vi "solar_visa VISA Query (Error).vi"(6 "ms Read Wait (0)":u32, 8 "error in (no error)":errorcluster, 9 "Bytes Expected (0 = 1024)":u32, 10 "Error Query (\"\" = No Query)":string, 11 "VISA Resource in":refnum<visa-resource-name>) -> (0 "error out":errorcluster, 3 "VISA Resource out":refnum<visa-resource-name>)   [LabVIEW 2018]
doc: "This queries instrument errors from the VISA session. By default, the error code integer is expected at the begining of the <b>Error Query</b> response (i.e \"+7: Invalid parameter...\"). To avoid an error lockout, the error query is limited to 100 errors. \nIf <b>Error in</b> contains a timeout error this clears the VISA buffer."
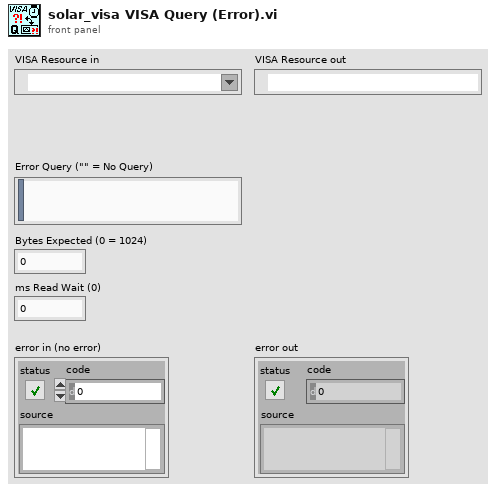
[diagram p1: front panel]
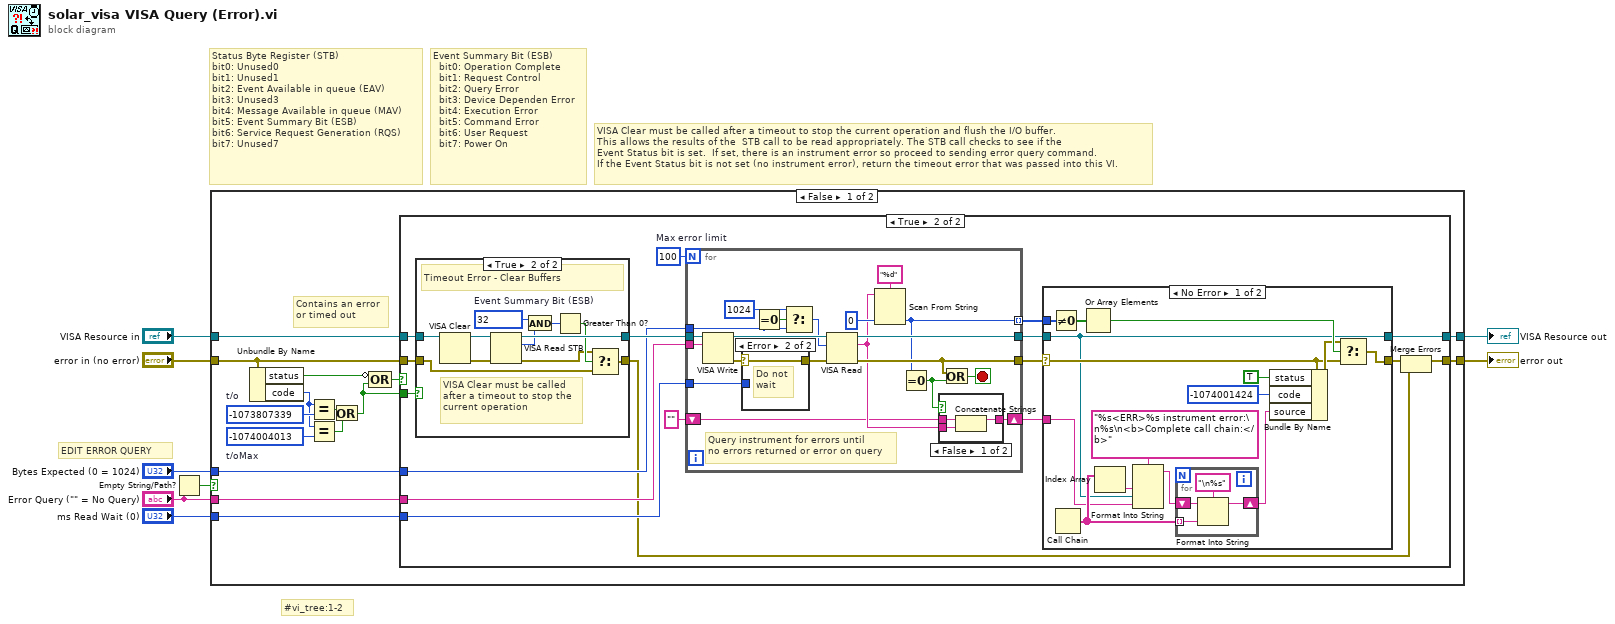
[diagram p0: block diagram]
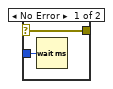
[diagram p5: hidden frame]
diagram:
  # "#vi_tree:1-2"
  # "EDIT ERROR QUERY"
  # "Event Summary Bit (ESB)\n  bit0: Operation Complete\n  bit1: Request Control\n  bit2: Query Error\n  bit3: Device Dependen Error\n  bit4: Execution Error\n  bit5: Command Error\n  bit6: User Request\n  bit7: Power On"
  # "VISA Clear must be called after a timeout to stop the current operation and flush the I/O buffer.\nThis allows the results of the  STB call to be read appropriately. The STB call checks to see if the \nEvent Status bit is set.  If set, there is an instrument error so proceed to sending error query command.  \nIf the Event Status bit is not set (no instrument error), return the timeout error that was passed into this VI."
  # "Status Byte Register (STB)\nbit0: Unused0\nbit1: Unused1\nbit2: Event Available in queue (EAV)\nbit3: Unused3\nbit4: Message Available in queue (MAV)\nbit5: Event Summary Bit (ESB)\nbit6: Service Request Generation (RQS)\nbit7: Unused7"
  n1 = Empty String/Path?(string/path="Error Query (\"\" = No Query)") -> (empty?=w1:bool)
  n2 = case shown="False" w1 {
    tunnel: "error in (no error)" -> [w12 w104]
    tunnel: "VISA Resource in" -> [w11 w105]
    tunnel: "Error Query (\"\" = No Query)" -> [w23 _]
    tunnel: "ms Read Wait (0)" -> [w22 _]
    tunnel: "Bytes Expected (0 = 1024)" -> [w21 _]
    tunnel: [w20 w105] -> w7
    tunnel: [w19 w104] -> w2
    frame False {
      w15 = -1074004013  # t/oMax
      w17 = -1073807339  # t/o
      # "Contains an error\nor timed out"
      n3 = Unbundle By Name(w12) -> ("status"=w18:bool, "code"=w13:i32)
      n4 = Equal?(x=w13, y=w17) -> (x = y?=w16:bool)
      n5 = Equal?(x=w13, y=w15) -> (x = y?=w14:bool)
      n6 = Or(x=w16, y=w14) -> (x .or. y?=w10:bool)
      n7 = Compound Arithmetic op=OR(invert w18, w10) -> (w9:bool)
      n8 = case shown="True" w9 {
        tunnel: w23 -> [_ w42]
        tunnel: w22 -> [_ w41]
        tunnel: w21 -> [_ w36]
        tunnel: [w25 w31] -> w20
        tunnel: [w24 w28] -> w19
        tunnel: w12 -> [w24 w40]
        tunnel: w11 -> [w25 w39]
        tunnel: w10 -> [_ w37]
        frame False {
        }
        frame True {
          w35 = 100  # Max error limit
          n9 = case shown="True" w37 {
            tunnel: w39 -> [w91 w103]
            tunnel: [w91 w101] -> w38
            tunnel: w40 -> [w92 w94]
            tunnel: [w92 w93] -> w27
            frame False {
            }
            frame True {
              w98 = u16 32  # Event Summary Bit (ESB)
              # "VISA Clear must be called\nafter a timeout to stop the\ncurrent operation"
              # "Timeout Error - Clear Buffers"
              n10 = VISA Clear(VISA resource name=w103) -> (VISA resource name out=w102:refnum<visa-resource-name>, error out=w100:errorcluster)  [unwired: 1 in]
              n11 = VISA Read STB(8:w100, 11:w102) -> (0:w95:errorcluster, 2:w99:u16, 3:w101:refnum<visa-resource-name>)
              n12 = And(x=w98, y=w99) -> (x .and. y?=w97:u16)
              n13 = Greater Than 0?(x=w97) -> (x > 0?=w96:bool)
              n14 = Select(t=w95, s=w96, f=w94) -> (s? t:f=w93:errorcluster)
            }
          }
          n15 = for {
            N: w35 -> [_]
            tunnel: w42 -> [w83]
            tunnel: w41 -> [w82]
            tunnel: [w71] -> w33
            tunnel: w36 -> [w74]
            tunnel: w38 -> [w77]
            tunnel: [w78] -> w30
            tunnel: [w67] -> w26 mode=indexing
            shift-right: [w68] -> w32
            shift-left: "" -> [w66]
            stop <- w70 stop-if-true
            # "Query instrument for errors until\nno errors returned or error on query"
            n16 = VISA Write(VISA resource name=w77, write buffer=w83) -> (VISA resource name out=w79:refnum<visa-resource-name>, error out=w80:errorcluster)  [unwired: 1 in, 1 out]
            n17 = case shown="Error" w80 {
              tunnel: w82 -> [w89 _]
              tunnel: [w88 w90] -> w81
              selector: w80 -> [w88 w90]
              frame No Error {
                n18 = Wait (ms)(milliseconds to wait=w89) -> ()  [unwired: 1 out]
              }
              frame Error {
                # "Do not\nwait"
              }
            }
            n19 = Equal To 0?(x=w74) -> (x = 0?=w76:bool)
            n20 = Select(t=u32 1024, s=w76, f=w74) -> (s? t:f=w73:u32)
            n21 = VISA Read(VISA resource name=w79, byte count=w73, error in (no error)=w81) -> (VISA resource name out=w78:refnum<visa-resource-name>, read buffer=w69:string, error out=w71:errorcluster)  [unwired: 1 out]
            n22 = Scan From String(format string="%d" ("t"), input string=w69, default 1=i64 0 ("default value 1")) -> (output 1=w67:i64)  [unwired: 2 in, 3 out]
            n23 = Equal To 0?(x=w67) -> (x = 0?=w65:bool)
            n24 = case shown="False" w65 {
              tunnel: w69 -> [w86 _]
              tunnel: [w85 w87] -> w68
              tunnel: w66 -> [w84 w87]
              frame False {
                n25 = Concatenate Strings(w84, w86) -> (w85:string)
              }
              frame True {
              }
            }
            n26 = Or(x=w71, y=w65) -> (x .or. y?=w70:bool)
          }
          n27 = case shown="No Error" w33 {
            selector: w33 -> [w52 w63]
            tunnel: w32 -> [w44 _]
            tunnel: [w57 w63] -> w29
            tunnel: w26 -> [w56 _]
            tunnel: [w45 w62] -> w31
            tunnel: w30 -> [w45 w62]
            frame No Error {
              n28 = Not Equal To 0?(x=w56) -> (x != 0?=w55:bool[])
              n29 = Call Chain() -> (call chain=w46:string[])
              n30 = Or Array Elements(Boolean array=w55) -> (logical OR=w54:bool)
              n31 = Index Array(array=w46) -> (element=w48:string)  [unwired: 1 in]
              n32 = Format Into String(format string="%s<ERR>%s instrument error:\n%s\n<b>Complete call chain:</b>", w48, w45, w44) -> (resulting string=w47:string)  [unwired: 2 in, 1 out]
              n33 = for {
                tunnel: w46 -> [w61] mode=indexing
                shift-right: [w60] -> w43
                shift-left: w47 -> [w59]
                n34 = Format Into String(format string="\n%s", initial string=w59, w61) -> (resulting string=w60:string)  [unwired: 1 in, 1 out]
              }
              n35 = Bundle By Name(cluster=w52, "status"=TRUE, "code"=-1074001424 ("Code"), "source"=w43) -> (w53:errorcluster)
              n36 = Select(t=w53, s=w54, f=w52) -> (s? t:f=w57:errorcluster)
            }
            frame Error {
              # "IO Error"
            }
          }
          n37 = Merge Errors(w29, w27) -> (w28:errorcluster)
        }
      }
    }
    frame True {
      # "No error query defined\n- Do nothing"
    }
  }
  "error out" <- w2
  "VISA Resource out" <- w7
